vi "Read Plugin Settings ID.vi"(8 "error in (no error)":errorcluster, 10 "Plugin ID":string, 11 "Configuration Session in":refnum<class "Configuration Session.lvclass">) -> (0 "error out":errorcluster, 1 "Settings ID":string, 3 "Configuration Session out":refnum<class "Configuration Session.lvclass">, 4 "found?":bool)   [LabVIEW 2017, in "DSF Core.lvlib" / "Configuration Session.lvclass"]
uses:
  Configuration Session.lvclass
  Configuration Session.lvclass/Configuration Session.ctl
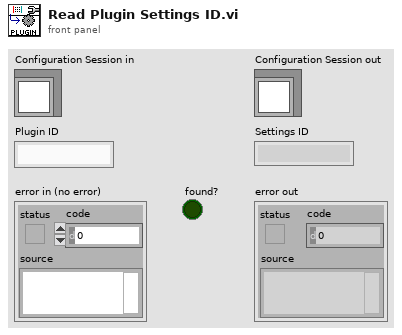
[diagram p1: front panel]
types:
  T1 = typedef "DSF Core.lvlib/Configuration Session.lvclass/DSF Config Data Ref.ctl" = refnum<data-value>
  T2 = typedef "DSF Core.lvlib/Configuration Session.lvclass/DSF Config Data.ctl" = cluster{"dsf configuration":T3, "path":path, "dirty":bool}
  T3 = typedef "DSF Core.lvlib/Configuration Session.lvclass/Internal.DSF Configuration.ctl" = cluster{"dsfversion":T4, "version":T4, "plugins":T5[], "groups":T8[], "transfers":T10[], "channels":T12[], "settings":T14[]}
  T4 = typedef "DSF Version Info.ctl" = cluster{"major":u32, "minor":u32, "fix":u32, "build":string}
  T5 = typedef "DSF Core.lvlib/Configuration Session.lvclass/Internal.DSF Plugin with ID.ctl" = cluster{"id":string, "values":T6}
  T6 = typedef "DSF Core.lvlib/Configuration Session.lvclass/Internal.DSF Plugin Info.ctl" = cluster{"type":string, "timing":T7, "group ids":string[], "settings id":string}
  T7 = typedef "DSF Timing Info.ctl" = cluster{"priority":u64, "decimation":u64, "offset":u64}
  T8 = typedef "DSF Core.lvlib/Configuration Session.lvclass/Internal.DSF Group with ID.ctl" = cluster{"id":string, "values":T9}
  T9 = typedef "DSF Core.lvlib/Configuration Session.lvclass/Internal.DSF Group Info.ctl" = cluster{"direction":i32, "timing":T7, "transfer ids":string[], "settings id":string}
  T10 = typedef "DSF Core.lvlib/Configuration Session.lvclass/Internal.DSF Transfer with ID.ctl" = cluster{"id":string, "values":T11}
  T11 = typedef "DSF Core.lvlib/Configuration Session.lvclass/Internal.DSF Transfer Info.ctl" = cluster{"byte order":i32, "channel ids":string[], "settings id":string}
  T12 = typedef "DSF Core.lvlib/Configuration Session.lvclass/Internal.DSF Channel with ID.ctl" = cluster{"id":string, "values":T13}
  T13 = typedef "DSF Core.lvlib/Configuration Session.lvclass/Internal.DSF Channel Info.ctl" = cluster{"count":u64, "buffer offset":u64, "data type":i32, "settings id":string}
  T14 = typedef "DSF Core.lvlib/Configuration Session.lvclass/Internal.DSF Settings with ID.ctl" = cluster{"id":string, "values":T15}
  T15 = typedef "DSF Core.lvlib/Configuration Session.lvclass/Internal.DSF Settings Info.ctl" = cluster{"key":string, "value":string}[]
  T16 = typedef "DSF Core.lvlib/DSF Plugin Info.ctl" = cluster{"type":string, "timing":T17, "group ids":string[], "settings id":string}
  T17 = typedef "DSF Core.lvlib/DSF Timing Info.ctl" = cluster{"priority":u64, "decimation":u64, "offset":u64}
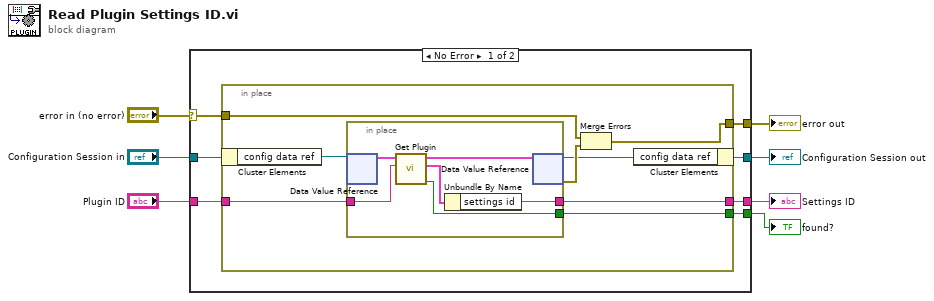
[diagram p0: block diagram]
diagram:
  n1 = case shown="No Error" "error in (no error)" {
    selector: "error in (no error)" -> [w14 w30]
    tunnel: "Configuration Session in" -> [w9 w29]
    tunnel: [w12 w30] -> w5
    tunnel: "Plugin ID" -> [w13 _]
    tunnel: [w11 _] -> w3
    tunnel: [w10 _] -> w2
    tunnel: [w8 w29] -> w1
    frame No Error {
      n2 = in-place {
        in-place-border: w14 -> [w15]
        in-place-border: w13 -> [w22]
        in-place-border: [w21] -> w12
        in-place-border: [w19] -> w11
        in-place-border: [w18] -> w10
        n3 = in-place-cluster #1(w9) -> ("config data ref"=w17:T1)
        n4 = in-place {
          in-place-border: w22 -> [w27]
          in-place-border: [w26] -> w19
          in-place-border: [w23] -> w18
          n5 = in-place-dvr #2(w17) -> (w28:T2)  [unwired: 1 out]
          n6 = call "Get Plugin.vi"("id"=w27, "DSF Configuration in"=w28) -> ("exists?"=w26:bool, "info"=w24:T16, "DSF Configuration out"=w25:T2)  [unwired: 6 in, 1 out]
          n7 = Unbundle By Name(w24) -> ("settings id"=w23:string)
          n8 = in-place-dvr #2(w25) -> (w16:T1, w20:errorcluster)
        }
        n9 = Merge Errors(w15, w20) -> (w21:errorcluster)
        n10 = in-place-cluster #1("config data ref"=w16) -> (w8:refnum<class "Configuration Session.lvclass">)
      }
    }
    frame Error {
    }
  }
  "error out" <- w5
  "found?" <- w3
  "Configuration Session out" <- w1
  "Settings ID" <- w2
